vi "Update Annotations.vi"(6 "Sample Period":dbl, 8 "Commands":T1(array[cluster]) {"System" items=["Elevator", "Carriage Intake STOP", "Carriage Intake RUN"]}, 9 "Trajectory Data":T3(array[cluster]), 10 "Robot Pt Index":i32) -> (2 "Velocity Trace":dbl[](array[numeric]), 3 "Annotation Data":T2(array[cluster]))   [LabVIEW 2020]
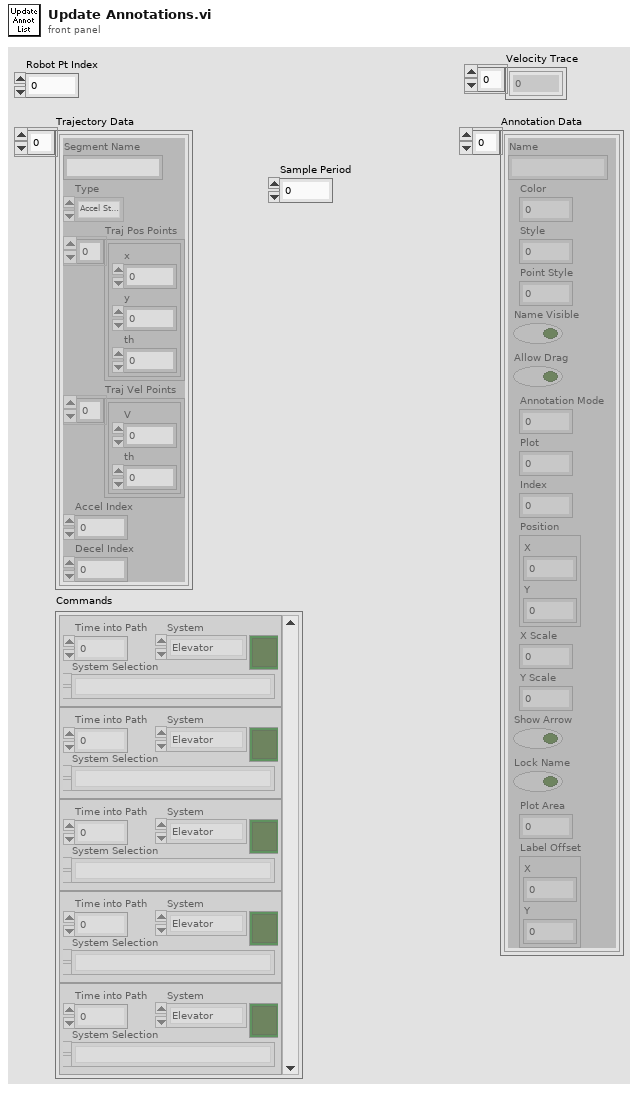
[diagram p1: front panel]
types:
  T1 = cluster{"Time into Path":dbl, "System":u16, "Item Selected?":bool, "System Selection":u16}[]
  T2 = cluster{"Name":string, "Color":u32, "Style":i32, "Point Style":i32, "Name Visible":bool, "Allow Drag":bool, "Annotation Mode":i32, "Plot":i32, "Index":i32, "Position":cluster{"X":dbl, "Y":dbl}, "X Scale":i32, "Y Scale":u32, "Show Arrow":bool, "Lock Name":bool, "Plot Area":i32, "Label Offset":cluster{"X":dbl, "Y":dbl}}[]
  T3 = cluster{"Segment Name":string, "Type":enum16{"Accel Straight", "Const Straight", "Blend", "Circle"}, "Traj Pos Points":cluster{"x":dbl, "y":dbl, "th":dbl}[], "Traj Vel Points":cluster{"V":dbl, "th":dbl}[], "Accel Index":i32, "Decel Index":i32}[]
  T4 = cluster{"Name":string, "Color":u32, "Style":i32, "Point Style":i32, "Name Visible":bool, "Allow Drag":bool, "Annotation Mode":i32, "Plot":i32, "Index":i32, "Position":cluster{"X":dbl, "Y":dbl}, "X Scale":i32, "Y Scale":u32, "Show Arrow":bool, "Lock Name":bool, "Plot Area":i32, "Label Offset":cluster{"X":dbl, "Y":i32}}
  T5 = enum16{"Accel Straight", "Const Straight", "Blend", "Circle"}
  T6 = cluster{"Name":string, "Color":u32, "Style":i32, "Point Style":i32, "Name Visible":bool, "Allow Drag":bool, "Annotation Mode":i32, "Plot":i32, "Index":i32, "Position":cluster{"X":dbl, "Y":dbl}, "X Scale":i32, "Y Scale":u32, "Show Arrow":bool, "Lock Name":bool, "Plot Area":i32, "Label Offset":cluster{"X":dbl, "Y":i32}}[]
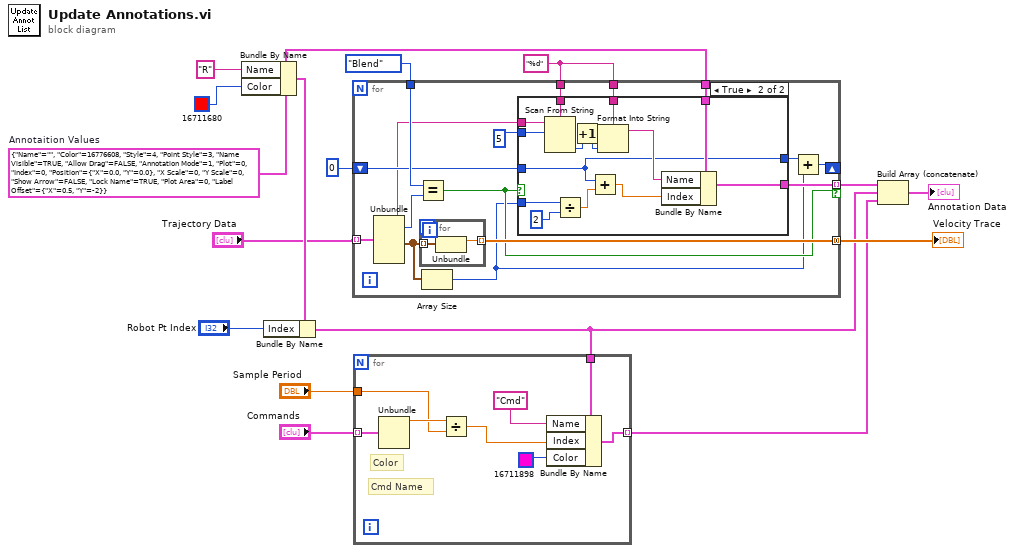
[diagram p0: block diagram]
diagram:
  w5 = T4 {"Name"="", "Color"=16776608, "Style"=4, "Point Style"=3, "Name Visible"=TRUE, "Allow Drag"=FALSE, "Annotation Mode"=1, "Plot"=0, "Index"=0, "Position"={"X"=0.0, "Y"=0.0}, "X Scale"=0, "Y Scale"=0, "Show Arrow"=FALSE, "Lock Name"=TRUE, "Plot Area"=0, "Label Offset"={"X"=0.5, "Y"=-2}}  # Annotaition Values
  w9 = "%d" ("Name")
  n1 = Bundle By Name(cluster=w5, "Name"="R", "Color"=u32 16711680) -> (w16:T4)
  n2 = Bundle By Name(cluster=w16, "Index"="Robot Pt Index") -> (w3:T4)
  n3 = for {
    tunnel: "Trajectory Data" -> [w32] mode=indexing
    tunnel: [w31] -> w6 mode=concatenating
    tunnel: T5."Blend" ("Type") -> [w30]
    shift-right: [w19] -> _
    shift-left: 0 -> [w27]
    tunnel: [w22] -> w11 mode=indexing if=w21
    tunnel: w5 -> [w26]
    tunnel: w9 -> [w24]
    tunnel: w9 -> [w23]
    n4 = Unbundle(w32) -> ("Segment Name"=w25:string, "Type"=w29:T5, "Traj Vel Points"=w28:cluster{"V":dbl, "th":dbl}[])  [unwired: 3 out]
    n5 = Equal?(x=w30, y=w29) -> (x = y?=w21:bool)
    n6 = for {
      tunnel: w28 -> [w49] mode=indexing
      tunnel: [w48] -> w31 mode=indexing
      n7 = Unbundle(w49) -> ("V"=w48:dbl)  [unwired: 1 out]
    }
    n8 = Array Size(array=w28) -> (size(s)=w18:i32)
    n9 = case shown="True" w21 {
      tunnel: w27 -> [w33 w41]
      tunnel: [w33 w41] -> w20
      tunnel: w26 -> [_ w47]
      tunnel: w25 -> [_ w46]
      tunnel: w24 -> [_ w45]
      tunnel: w23 -> [_ w44]
      tunnel: [_ w42] -> w22
      tunnel: w18 -> [_ w38]
      tunnel: 5 -> [_ w37]
      frame False {
      }
      frame True {
        n10 = Scan From String(format string=w45, input string=w46, initial scan location=w37) -> (output 1=w35:i32)  [unwired: 2 in, 3 out]
        n11 = Divide(x=w38, y=2) -> (x/y=w39:dbl)
        n12 = Increment(x=w35) -> (x+1=w34:i32)
        n13 = Add(x=w41, y=w39) -> (x+y=w36:dbl)
        n14 = Format Into String(format string=w44, w34) -> (resulting string=w43:string)  [unwired: 2 in, 1 out]
        n15 = Bundle By Name(cluster=w47, "Name"=w43, "Index"=w36) -> (w42:T4)
      }
    }
    n16 = Add(x=w20, y=w18) -> (x+y=w19:i32)
  }
  "Velocity Trace" <- w6
  n17 = for {
    tunnel: "Commands" -> [w57] mode=indexing
    tunnel: w3 -> [w56]
    tunnel: [w55] -> w1 mode=indexing
    tunnel: "Sample Period" -> [w52]
    # "Cmd Name"
    # "Color"
    n18 = Unbundle(w57) -> ("Time into Path"=w53:dbl)  [unwired: 3 out]
    n19 = Divide(x=w53, y=w52) -> (x/y=w51:dbl)
    n20 = Bundle By Name(cluster=w56, "Name"="Cmd", "Index"=w51, "Color"=u32 16711898) -> (w55:T4)
  }
  n21 = Build Array (concatenate)(w11, w3, w1) -> (→"Annotation Data":T6)
